vi "Keithley 2400 - Close.vi"(11 "Porta:":refnum<visa-resource-name>) -> ()   [LabVIEW 2019]
uses:
  <vilib>/Instr/_visa.llb/VISA Configure Serial Port (Instr).vi
panel:
  out "error out":errorcluster
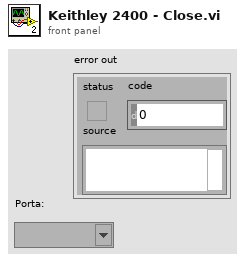
[diagram p1: front panel]
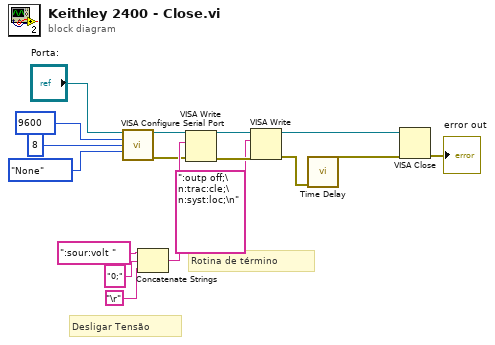
[diagram p0: block diagram]
diagram:
  # "Rotina de término"
  # "Desligar Tensão"
  n1 = call-poly "VISA Configure Serial Port"("VISA resource name"="Porta:", "baud rate (9600)"=u32 9600, "data bits (8)"=u16 8, "parity (0:none)"=enum16{"None", "Odd", "Even", "Mark", "Space"}."None") -> ("VISA resource name out"=w7:refnum<visa-resource-name>, "error out"=w6:errorcluster)  [unwired: 10 in]
  n2 = Concatenate Strings(":sour:volt " ("write buffer"), "0;" ("string"), "\r") -> (w15:string)
  n3 = VISA Write(VISA resource name=w7, write buffer=w15, error in (no error)=w6) -> (VISA resource name out=w14:refnum<visa-resource-name>, error out=w13:errorcluster)  [unwired: 1 out]
  n4 = VISA Write(VISA resource name=w14, write buffer=":outp off;\n:trac:cle;\n:syst:loc;\n", error in (no error)=w13) -> (VISA resource name out=w9:refnum<visa-resource-name>, error out=w8:errorcluster)  [unwired: 1 out]
  n5 = call "Time Delay"("error in (no error)"=w8) -> ("error out"=w1:errorcluster)  [unwired: 10 in]
  n6 = VISA Close(VISA resource name=w9, error in (no error)=w1) -> (error out=→"error out":errorcluster)
